vi "Create SuperProjectBaseActor.vi"(7 "Name":string, 8 "error in (no error)":errorcluster, 9 "Configuration":variant, 10 "ConfigManager":refnum<class "ConfigManager.lvclass">, 11 "SuperProjectBaseActor":refnum<class "SuperProjectBaseActor.lvclass">) -> (0 "error out":errorcluster, 3 "SuperProjectBaseActor out":refnum<class "SuperProjectBaseActor.lvclass">)   [LabVIEW 2014, in "SuperProjectBaseActor.lvclass"]
uses:
  SuperProjectBaseActor.lvclass
  <vilib>/LabVIEW Open Source/Configuration Manager/Manager/ConfigManager.lvclass
  ConfigurableActor/ConfigurableActor.lvclass/ConfigurableActor.ctl
  ConfigurableActor/ConfigurableActor.lvclass
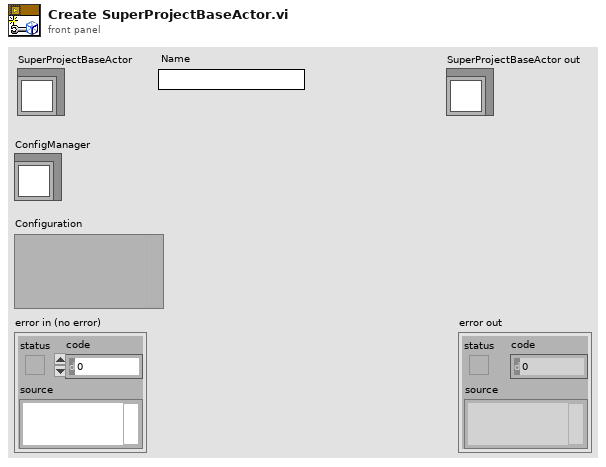
[diagram p1: front panel]
types:
  T1 = typedef "UniqueName.lvlib/NameRegistry.lvclass/RegistryConfiguration.ctl" = cluster{"Delimiter":refnum<class "Delimiter.lvclass">, "RandomStringGenerator":refnum<class "RandomStringGenerator.lvclass">, "UniquenessCriteria":refnum<class "UniquenessCriteria.lvclass">, "StringIncrement":refnum<class "StringIncrement.lvclass">}
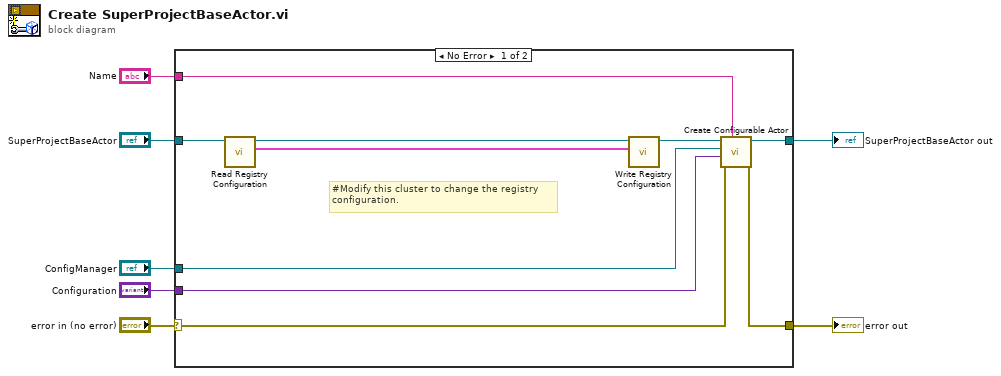
[diagram p0: block diagram]
diagram:
  n1 = case shown="No Error" "error in (no error)" {
    selector: "error in (no error)" -> [w12 w18]
    tunnel: "SuperProjectBaseActor" -> [w10 w19]
    tunnel: "ConfigManager" -> [w16 _]
    tunnel: [w17 w19] -> w5
    tunnel: [w11 w18] -> w3
    tunnel: "Name" -> [w14 _]
    tunnel: "Configuration" -> [w15 _]
    frame No Error {
      # "#Modify this cluster to change the registry\nconfiguration."
      n2 = call "Read Registry Configuration.vi"("ConfigurableActor in"=w10) -> ("Registry Configuration"=w8:T1, "ConfigurableActor out"=w9:refnum<class "SuperProjectBaseActor.lvclass">)  [unwired: 9 in]
      n3 = call "Write Registry Configuration.vi"("Registry Configuration"=w8, "ConfigurableActor in"=w9) -> ("ConfigurableActor out"=w13:refnum<class "SuperProjectBaseActor.lvclass">)  [unwired: 9 in]
      n4 = call "Create Configurable Actor.vi"("Name"=w14, "error in (no error)"=w12, "Configuration"=w15, "ConfigManager"=w16, "ConfigurableActor"=w13) -> ("error out"=w11:errorcluster, "ConfigurableActor out"=w17:refnum<class "SuperProjectBaseActor.lvclass">)  [unwired: 5 in]
    }
    frame Error {
    }
  }
  "SuperProjectBaseActor out" <- w5
  "error out" <- w3
